vi "Servidor-SAEG.vi"() -> (0 "error":i32, 1 "status":bool)   [LabVIEW 2016]
uses:
  <vilib>/Analysis/NI_AALPro.lvlib
panel:
  in  "amplitude":dbl=1.0 format="%0.2f"
  in  "frequency":dbl=10.0 format="%0.2f"
  in  "service name":string
  out "Waveform Chart":dbl[](graph)
  in  "stop":bool
  in  "signal type":T1(ring)
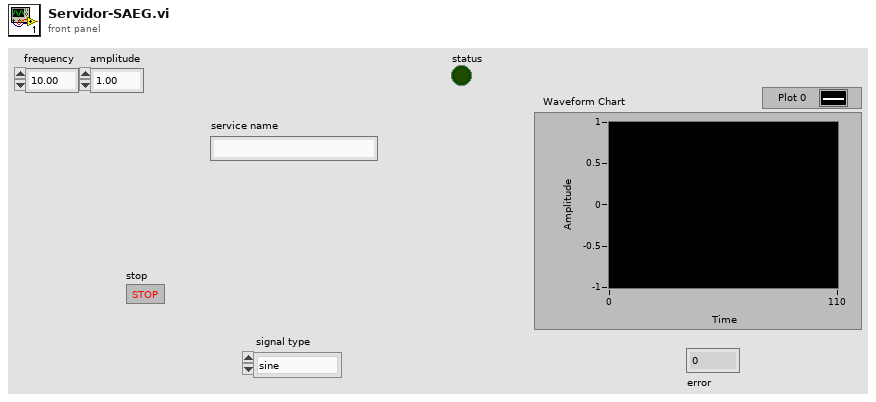
[diagram p1: front panel]
types:
  T1 = enum16{"sine", "cosine", "triangle", "square", "sawtooth", "increasing ramp", "decreasing ramp"}
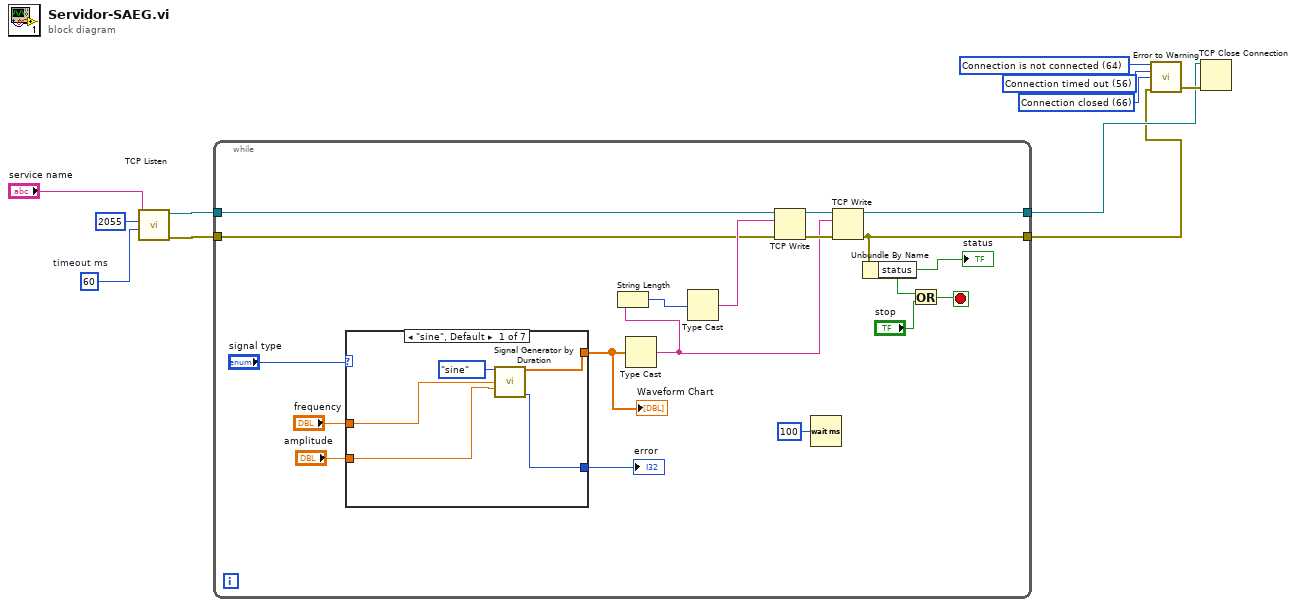
[diagram p0: block diagram]
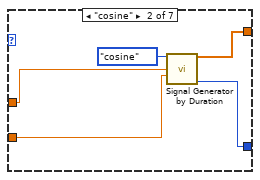
[diagram p2: hidden frame]
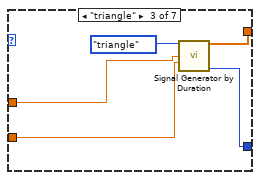
[diagram p3: hidden frame]
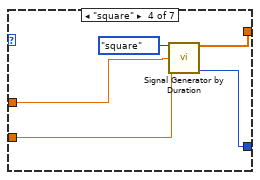
[diagram p4: hidden frame]
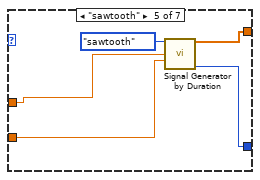
[diagram p5: hidden frame]
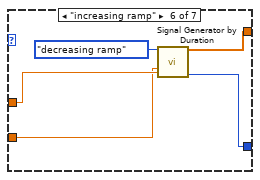
[diagram p6: hidden frame]
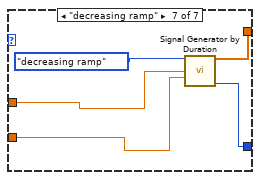
[diagram p7: hidden frame]
diagram:
  w4 = 56 items=["No Error", "Argument Error", "Memory Full", "Out of Zone", "End of File", "File Already Open", "Generic File IO Error", "File Not Found", "File Permission Error", "Disk Full", "Duplicate Path", "Too Many Files Open", "Not Enabled", "Resource File Not Found", "Cannot Add Resource", "Resource Not Found", "Image Not Found", "Image Memory Error", "Pen Does Not Exist", "Config Bad Type", "Config Token Not Found", "Config Parse Error", "Config Memory Error", "Bad External Code Format", "Bad External Code Offset", "External Code Not Present", "Null Window", "Destroy Window Mixup", "Null Menu", "Print Aborted", "Bad Print Record", "Print Driver Error", "Windows Error During Print", "Memory Error During Print", "Print Dialog Error", "Generic Print Error", "Invalid Device Refnum", "Device Not Found", "Device Parameter Error", "Device Unit Error", "Can't Open Device", "Device Call Aborted", "Generic Error", "Cancelled By User", "Object ID Too Low", "Object ID Too High", "Object Not In Heap", "Unknown Heap", "Bad DefProc ID", "DefProc Not In Table", "Message Out Of Range", "Null Method", "Unknown Message", "Manager Call Not Supported", "Bad address", "Connection In progress", "Connection timed out", "Connection is already in progress", "Network attribute not supported", "Network error", "Address in use", "System out of memory", "Connection aborted", "Connection refused", "Connection is not connected", "Connection is already connected", "Connection closed", "Initialize error (interapplication manager)", "Bad occurrence", "Wait on unbound occurrence handler", "Occurrence queue overflow", "Bad path", "Semaphore not signaled", "Unrecognized type (interapplication manager)"] ("2nd Error to Convert")
  w5 = 66 items=["No Error", "Argument Error", "Memory Full", "Out of Zone", "End of File", "File Already Open", "Generic File IO Error", "File Not Found", "File Permission Error", "Disk Full", "Duplicate Path", "Too Many Files Open", "Not Enabled", "Resource File Not Found", "Cannot Add Resource", "Resource Not Found", "Image Not Found", "Image Memory Error", "Pen Does Not Exist", "Config Bad Type", "Config Token Not Found", "Config Parse Error", "Config Memory Error", "Bad External Code Format", "Bad External Code Offset", "External Code Not Present", "Null Window", "Destroy Window Mixup", "Null Menu", "Print Aborted", "Bad Print Record", "Print Driver Error", "Windows Error During Print", "Memory Error During Print", "Print Dialog Error", "Generic Print Error", "Invalid Device Refnum", "Device Not Found", "Device Parameter Error", "Device Unit Error", "Can't Open Device", "Device Call Aborted", "Generic Error", "Cancelled By User", "Object ID Too Low", "Object ID Too High", "Object Not In Heap", "Unknown Heap", "Bad DefProc ID", "DefProc Not In Table", "Message Out Of Range", "Null Method", "Unknown Message", "Manager Call Not Supported", "Bad address", "Connection In progress", "Connection timed out", "Connection is already in progress", "Network attribute not supported", "Network error", "Address in use", "System out of memory", "Connection aborted", "Connection refused", "Connection is not connected", "Connection is already connected", "Connection closed", "Initialize error (interapplication manager)", "Bad occurrence", "Wait on unbound occurrence handler", "Occurrence queue overflow", "Bad path", "Semaphore not signaled", "Unrecognized type (interapplication manager)"] ("3rd Error to Convert")
  w6 = 64 items=["No Error", "Argument Error", "Memory Full", "Out of Zone", "End of File", "File Already Open", "Generic File IO Error", "File Not Found", "File Permission Error", "Disk Full", "Duplicate Path", "Too Many Files Open", "Not Enabled", "Resource File Not Found", "Cannot Add Resource", "Resource Not Found", "Image Not Found", "Image Memory Error", "Pen Does Not Exist", "Config Bad Type", "Config Token Not Found", "Config Parse Error", "Config Memory Error", "Bad External Code Format", "Bad External Code Offset", "External Code Not Present", "Null Window", "Destroy Window Mixup", "Null Menu", "Print Aborted", "Bad Print Record", "Print Driver Error", "Windows Error During Print", "Memory Error During Print", "Print Dialog Error", "Generic Print Error", "Invalid Device Refnum", "Device Not Found", "Device Parameter Error", "Device Unit Error", "Can't Open Device", "Device Call Aborted", "Generic Error", "Cancelled By User", "Object ID Too Low", "Object ID Too High", "Object Not In Heap", "Unknown Heap", "Bad DefProc ID", "DefProc Not In Table", "Message Out Of Range", "Null Method", "Unknown Message", "Manager Call Not Supported", "Bad address", "Connection In progress", "Connection timed out", "Connection is already in progress", "Network attribute not supported", "Network error", "Address in use", "System out of memory", "Connection aborted", "Connection refused", "Connection is not connected", "Connection is already connected", "Connection closed", "Initialize error (interapplication manager)", "Bad occurrence", "Wait on unbound occurrence handler", "Occurrence queue overflow", "Bad path", "Semaphore not signaled", "Unrecognized type (interapplication manager)"] ("1st Error to Convert")
  w11 = 60  # timeout ms
  n1 = call <vilib>:"TCP Listen.vi"("timeout ms (wait forever: -1)"=w11, "port"=u16 2055 ("Porta"), "service name"="service name") -> ("error out"=w8:errorcluster, "connection ID"=w9:refnum<k5>)  [unwired: 4 in, 3 out]
  n2 = while {
    tunnel: w9 -> [w26]
    tunnel: w8 -> [w13]
    tunnel: [w14] -> w1
    tunnel: [w20] -> w2
    stop <- w22 stop-if-true
    n3 = case shown="\"sine\", Default" "signal type" {
      tunnel: [w34 w39 w44 w49 w54 w59 w64] -> w16
      tunnel: "frequency" -> [w32 w37 w42 w47 w51 w57 w62]
      tunnel: "amplitude" -> [w31 w36 w41 w46 w52 w56 w61]
      tunnel: [w30 w35 w40 w45 w50 w55 w60] -> w12
      frame "sine", Default {
        n4 = call <vilib>:"Signal Generator by Duration.vi"("signal type"=T1."sine", "frequency"=w32, "amplitude"=w31) -> ("signal"=w34:dbl[], "error"=w30:i32)  [unwired: 9 in, 2 out]
      }
      frame "cosine" {
        n5 = call <vilib>:"Signal Generator by Duration.vi"("signal type"=T1."cosine", "frequency"=w37, "amplitude"=w36) -> ("signal"=w39:dbl[], "error"=w35:i32)  [unwired: 9 in, 2 out]
      }
      frame "triangle" {
        n6 = call <vilib>:"Signal Generator by Duration.vi"("signal type"=T1."triangle", "frequency"=w42, "amplitude"=w41) -> ("signal"=w44:dbl[], "error"=w40:i32)  [unwired: 9 in, 2 out]
      }
      frame "square" {
        n7 = call <vilib>:"Signal Generator by Duration.vi"("signal type"=T1."square", "frequency"=w47, "amplitude"=w46) -> ("signal"=w49:dbl[], "error"=w45:i32)  [unwired: 9 in, 2 out]
      }
      frame "sawtooth" {
        n8 = call <vilib>:"Signal Generator by Duration.vi"("signal type"=T1."sawtooth", "frequency"=w51, "amplitude"=w52) -> ("signal"=w54:dbl[], "error"=w50:i32)  [unwired: 9 in, 2 out]
      }
      frame "increasing ramp" {
        n9 = call <vilib>:"Signal Generator by Duration.vi"("signal type"=T1."decreasing ramp", "frequency"=w57, "amplitude"=w56) -> ("signal"=w59:dbl[], "error"=w55:i32)  [unwired: 9 in, 2 out]
      }
      frame "decreasing ramp" {
        n10 = call <vilib>:"Signal Generator by Duration.vi"("signal type"=T1."decreasing ramp", "frequency"=w62, "amplitude"=w61) -> ("signal"=w64:dbl[], "error"=w60:i32)  [unwired: 9 in, 2 out]
      }
    }
    "Waveform Chart" <- w16
    "error" <- w12
    n11 = Type Cast(x=w16) -> (*(type *) &x=w24:string)  [unwired: 1 in]
    n12 = String Length(string=w24) -> (length=w28:i32)
    n13 = Type Cast(x=w28) -> (*(type *) &x=w27:string)  [unwired: 1 in]
    n14 = TCP Write(connection ID=w26, data in=w27, error in (no error)=w13) -> (connection ID out=w29:refnum<k5>, error out=w25:errorcluster)  [unwired: 1 in, 1 out]
    n15 = Wait (ms)(milliseconds to wait=u32 100) -> ()  [unwired: 1 out]
    n16 = TCP Write(connection ID=w29, data in=w24, error in (no error)=w25) -> (connection ID out=w20:refnum<k5>, error out=w14:errorcluster)  [unwired: 1 in, 1 out]
    n17 = Unbundle By Name(w14) -> ("status"=w15:bool)
    "status" <- w15
    n18 = Or(x=w15, y="stop") -> (x .or. y?=w22:bool)
  }
  n19 = call <vilib>:"Error to Warning.vi"("1st Error to Convert"=w6, "2nd Error to Convert"=w4, "3rd Error to Convert"=w5, "error in"=w1) -> ("warning out"=w3:errorcluster)  [unwired: 11 in]
  n20 = TCP Close Connection(connection ID=w2, error in (no error)=w3) -> ()  [unwired: 1 in, 2 out]
